vi "ELVIS III v1.0 Configure DO DIR.vi"(7 "Apply Bitmask?":bool=TRUE, 8 "error in (no error)":errorcluster, 10 "Bitmask Array":bool[][](array[boolean]), 11 "myRIO FPGA Ref In":T1) -> (0 "error out":errorcluster)   [LabVIEW 2021]
uses:
  <vilib>/myRIO/Common/Instrument Driver Framework/Utilities/typedefs/Generic FPGA Reference.ctl
  <vilib>/myRIO/Common/Instrument Driver Framework/ELVIS III v1.0/DO Block/typedefs/ELVIS III DO Block FPGA Reference.ctl
  <vilib>/myRIO/Common/Instrument Driver Framework/ELVIS III v1.0/Resource Manager/typedefs/ELVIS III v1.0 Connector List.ctl
  <vilib>/Utility/error.llb/Error Cluster From Error Code.vi
  <vilib>/rvi/errors/niLvFpgaAdjustHostInterfaceError.vi
  <vilib>/rvi/interface/nirviReadWriteControl/nirviReadWriteControl.xnode
  NiFpgaLv.dll
  <vilib>/rvi/interface/Simulation/niFpgaSimulationCallBeginRW.vi
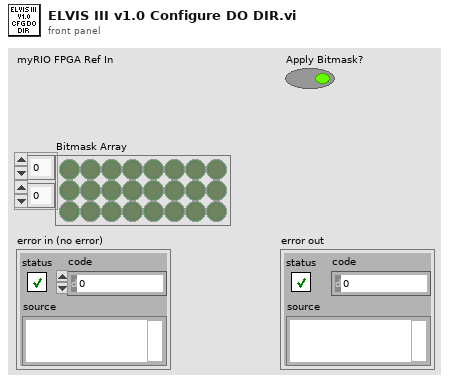
[diagram p1: front panel]
types:
  T1 = typedef "Generic FPGA Reference.ctl" = refnum<k20>
  T2 = typedef "ELVIS III DO Block FPGA Reference.ctl" = refnum<k20>
  T3 = typedef "ELVIS III v1.0 Connector List.ctl" = enum32{"None", "ConnectorA", "ConnectorB"}
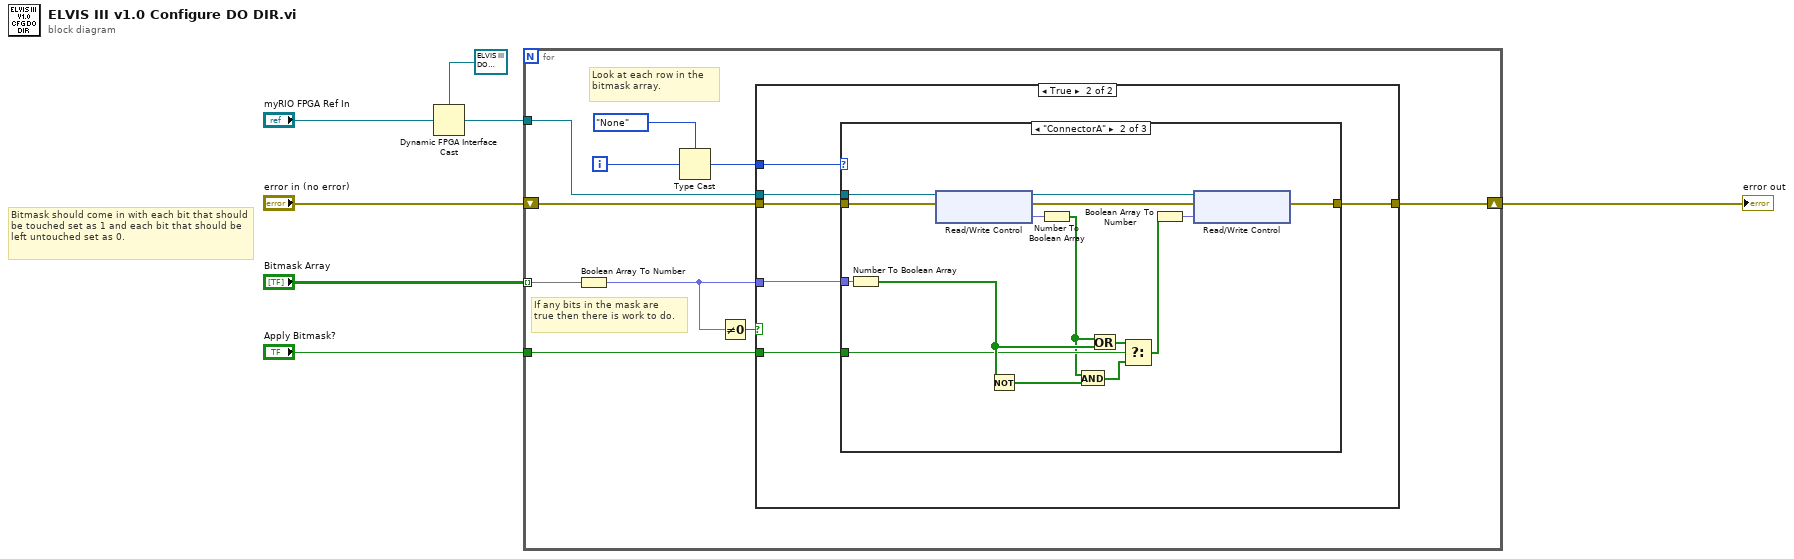
[diagram p0: block diagram]
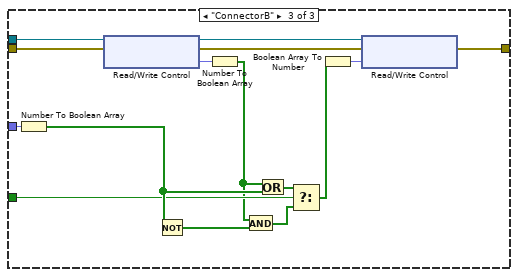
[diagram p4: hidden frame]
diagram:
  # "Bitmask should come in with each bit that should be touched set as 1 and each bit that should be left untouched set as 0."
  n1 = Dynamic FPGA Interface Cast(Session In=T2 refnum ("FPGA Interface"), Type="myRIO FPGA Ref In") -> (Session Out=w4:T2)
  n2 = for {
    tunnel: w4 -> [w15]
    tunnel: "Bitmask Array" -> [w11] mode=indexing
    tunnel: "Apply Bitmask?" -> [w14]
    shift-right: [w16] -> w6
    shift-left: "error in (no error)" -> [w17]
    i -> [w8]
    # "Look at each row in the bitmask array."
    # "If any bits in the mask are\ntrue then there is work to do."
    n3 = Boolean Array To Number(Boolean array=w11) -> (number=w13:fxp<+,20,20>)
    n4 = Type Cast(type=ELVIS_III_v1.0_Connector_List."None" ("Connector List"), x=w8) -> (*(type *) &x=w9:T3)
    n5 = Not Equal To 0?(x=w13) -> (x != 0?=w12:bool)
    n6 = case shown="True" w12 {
      tunnel: w15 -> [_ w24]
      tunnel: w17 -> [w18 w23]
      tunnel: [w18 w22] -> w16
      tunnel: w13 -> [_ w21]
      tunnel: w14 -> [_ w20]
      tunnel: w9 -> [_ w19]
      frame False {
        # "There are no bits to change for this connector."
      }
      frame True {
        n7 = case shown="\"ConnectorA\"" w19 {
          tunnel: w24 -> [_ w39 w54]
          tunnel: w23 -> [w25 w40 w55]
          tunnel: [w25 w38 w53] -> w22
          tunnel: w21 -> [_ w35 w50]
          tunnel: w20 -> [_ w36 w51]
          frame "None", Default {
            # "Do Nothing"
          }
          frame "ConnectorA" {
            n8 = Number To Boolean Array(number=w35) -> (Boolean array=w37:bool[])
            n9 = xnode "Read/Write Control"("FPGA VI Reference In"=w39, "error in"=w40) -> ("FPGA VI Reference Out"=w33:T2, "error out"=w34:errorcluster, "DIO.A_19:0.DIR"=w27:fxp<+,20,20>)
            n10 = Not(x=w37) -> (.not. x?=w29:bool[])
            n11 = Number To Boolean Array(number=w27) -> (Boolean array=w31:bool[])
            n12 = And(x=w31, y=w29) -> (x .and. y?=w30:bool[])
            n13 = Or(x=w31, y=w37) -> (x .or. y?=w28:bool[])
            n14 = Select(t=w28, s=w36, f=w30) -> (s? t:f=w32:bool[])
            n15 = Boolean Array To Number(Boolean array=w32) -> (number=w26:fxp<+,20,20>)
            n16 = xnode "Read/Write Control"("FPGA VI Reference In"=w33, "error in"=w34, "DIO.A_19:0.DIR"=w26) -> ("error out"=w38:errorcluster)  [unwired: 1 out]
          }
          frame "ConnectorB" {
            n17 = Number To Boolean Array(number=w50) -> (Boolean array=w52:bool[])
            n18 = xnode "Read/Write Control"("FPGA VI Reference In"=w54, "error in"=w55) -> ("FPGA VI Reference Out"=w48:T2, "error out"=w49:errorcluster, "DIO.B_19:0.DIR"=w42:fxp<+,20,20>)
            n19 = Not(x=w52) -> (.not. x?=w44:bool[])
            n20 = Number To Boolean Array(number=w42) -> (Boolean array=w46:bool[])
            n21 = And(x=w46, y=w44) -> (x .and. y?=w45:bool[])
            n22 = Or(x=w46, y=w52) -> (x .or. y?=w43:bool[])
            n23 = Select(t=w43, s=w51, f=w45) -> (s? t:f=w47:bool[])
            n24 = Boolean Array To Number(Boolean array=w47) -> (number=w41:fxp<+,20,20>)
            n25 = xnode "Read/Write Control"("FPGA VI Reference In"=w48, "error in"=w49, "DIO.B_19:0.DIR"=w41) -> ("error out"=w53:errorcluster)  [unwired: 1 out]
          }
        }
      }
    }
  }
  "error out" <- w6
